vi "ReadSerial_and_Plot_Basic_JE_002.vi"() -> ()   [LabVIEW 2011]
uses:
  <vilib>/Instr/_visa.llb/VISA Configure Serial Port (Serial Instr).vi
panel:
  in  "N data blocks to read":dbl=1.0
  in  "byte order (0:big-endian, network order) 2":T1(ring)
  out "Nbytes written from Teensy to Serial Port":u32
  out "strlen":i32
  in  "byte order (0:big-endian, network order)":T1(ring)
  out "Graphical Representation of 1-D Data Stream":u16[](graph)
  out "concatenated string":string
  out "ascii code u8":i32
  out "Waveform Chart for 32 Chans":T2(graph)
  out "size(s)":i32
  in  "stop":bool
  in  "VISA resource name":refnum<visa-resource-name>
  in  "baud rate (9600)":u32=9600
  in  "data bits (8)":u16=8 min=5 max=8 step=1
  in  "stop bits (10: 1 bit)":u16(ring)=10 items=["1.0"=10, "1.5"=15, "2.0"=20]
  in  "flow control (0:none)":u16(ring) items=["None", "XON/XOFF", "RTS/CTS", "XON/XOFF & RTS/CTS", "DTR/DSR", "XON/XOFF & DTR/DSR"]
  in  "parity (0:none)":enum16{"None", "Odd", "Even", "Mark", "Space"}(ring)
  in  "file (use dialog)":path
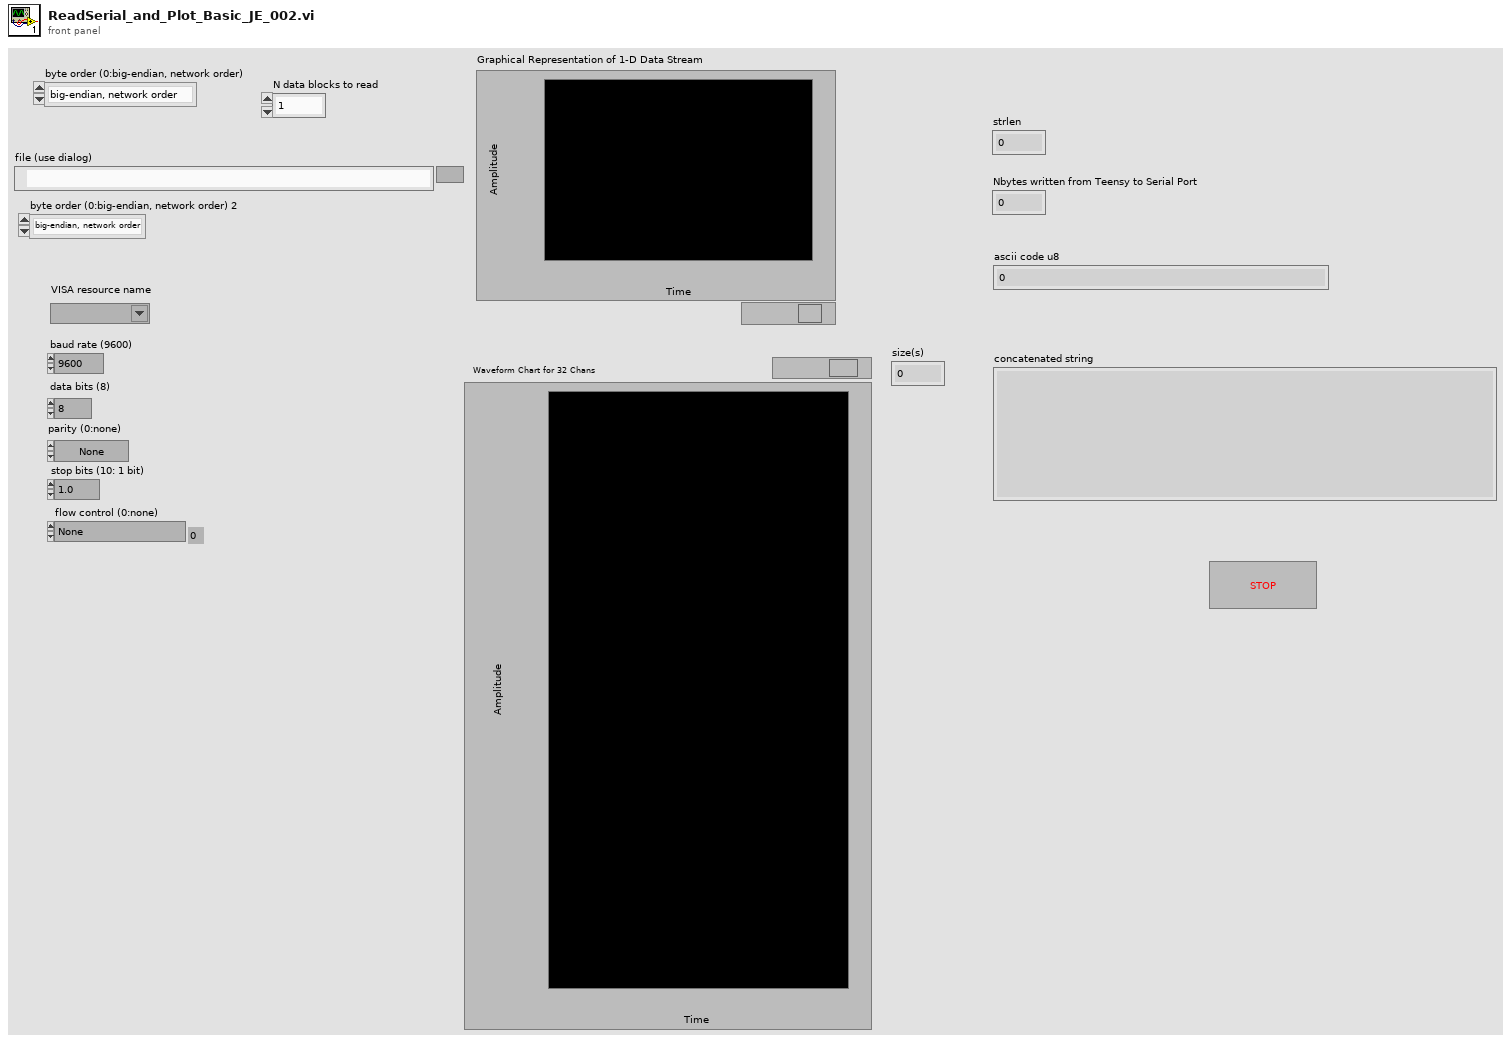
[diagram p1: front panel]
types:
  T1 = enum16{"big-endian, network order", "native, host order", "little-endian"}
  T2 = cluster{"[0]":u16, "[1]":u16, "[2]":u16, "[3]":u16, "[4]":u16, "[5]":u16, "[6]":u16, "[7]":u16, "[8]":u16, "[9]":u16, "[10]":u16, "[11]":u16, "[12]":u16, "[13]":u16, "[14]":u16, "[15]":u16, "[16]":u16, "[17]":u16, "[18]":u16, "[19]":u16, "[20]":u16, "[21]":u16, "[22]":u16, "[23]":u16, "[24]":u16, "[25]":u16, "[26]":u16, "[27]":u16, "[28]":u16, "[29]":u16, "[30]":u16, "[31]":u16}
  T3 = enum16{"open", "replace", "create", "open or create", "replace or create", "replace or create with confirmation"}
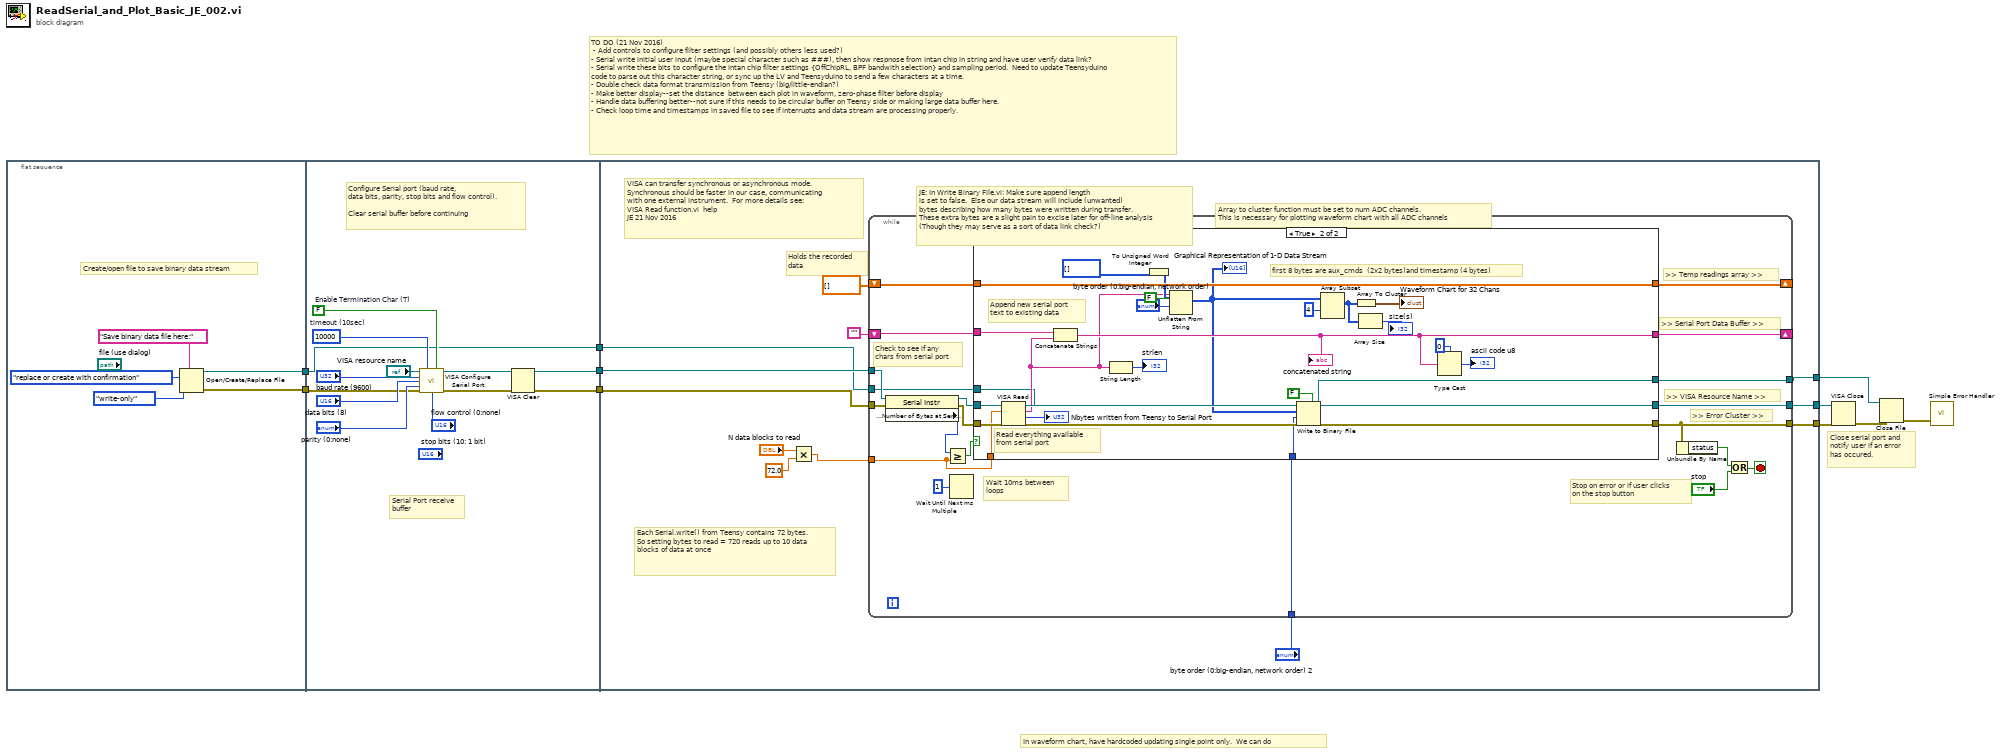
[diagram p0: block diagram]
diagram:
  # "TO DO (21 Nov 2016)\n - Add controls to configure filter settings (and possibly others less used?)\n- Serial write initial user input (maybe special character such as ###), then show respnose from Intan chip in string and have user verify data link?\n- Serial write these bits to configure the Intan chip filter settings {OffChipRL, BPF bandwith selection} and sampling period.  Need to update Teensyduino code to parse out this character string, or sync up the LV and Teensyduino to send a few characters at a time. \n- Double check data format transmission from Teensy (big/little-endian?)\n- Make better display--set the distance  between each plot in waveform, zero-phase filter before display\n- Handle data buffering better--not sure if this needs to be circular buffer on Teensy side or making large data buffer here.\n- Check loop time and timestamps in saved file to see if interrupts and data stream are processing properly."
  # "In waveform chart, have hardcoded updating single point only.  We can do"
  # "Close serial port and\nnotify user if an error\nhas occured."
  n1 = flat-sequence {
    tunnel: [w12] -> w10
    tunnel: [w11] -> w2
    tunnel: w10 -> [w19]
    tunnel: [w18] -> w4
    tunnel: [w17] -> w3
    tunnel: w2 -> [w16]
    tunnel: [w16] -> w1
    tunnel: [w34] -> w7
    tunnel: [w33] -> w6
    tunnel: [w32] -> w5
    tunnel: w4 -> [w31]
    tunnel: w3 -> [w30]
    tunnel: w1 -> [w29]
    frame #0 {
      # "Create/open file to save binary data stream"
      n2 = Open/Create/Replace File(prompt="Save binary data file here:" ("prompt (Choose or enter file path)"), operation (0:open)=T3."replace or create with confirmation", access (0:read/write)=enum16{"read/write", "read-only", "write-only"}."write-only") -> (refnum out=w11:refnum<file>, error out=w12:errorcluster)  [unwired: 3 in, 1 out]
    }
    frame #1 {
      w27 = FALSE  # Enable Termination Char (T)
      w28 = u32 10000  # timeout (10sec)
      # "Configure Serial port (baud rate,\ndata bits, parity, stop bits and flow control).\n\nClear serial buffer before continuing"
      # "Serial Port receive\nbuffer"
      n3 = call-poly "VISA Configure Serial Port"("VISA resource name"="VISA resource name", "timeout (10sec)"=w28, "Enable Termination\nChar (T)"=w27, "baud rate (9600)"="baud rate (9600)", "data bits (8)"="data bits (8)", "parity (0:none)"="parity (0:none)", "error in (no error)"=w19, "flow control (0:none)"="flow control (0:none)") -> ("VISA resource name out"=w25:refnum<visa-resource-name>, "error out"=w26:errorcluster)  [unwired: 6 in]
      n4 = VISA Clear(VISA resource name=w25, error in (no error)=w26) -> (VISA resource name out=w18:refnum<visa-resource-name>, error out=w17:errorcluster)
    }
    frame #2 {
      # "Holds the recorded\ndata"
      # "Each Serial.write() from Teensy contains 72 bytes.  So setting bytes to read = 720 reads up to 10 data blocks of data at once"
      # "Array to cluster function must be set to num ADC channels. \nThis is necessary for plotting waveform chart with all ADC channels"
      # "JE: In Write Binary File.vi: Make sure append length \nis set to false.  Else our data stream will include (unwanted)\nbytes describing how many bytes were written during transfer.\nThese extra bytes are a slight pain to excise later for off-line analysis\n(Though they may serve as a sort of data link check?)"
      # "VISA can transfer synchronous or asynchronous mode.\nSynchronous should be faster in our case, communicating\nwith one external instrument.  For more details see: \nVISA Read function.vi  help \nJE 21 Nov 2016"
      n5 = Multiply(x="N data blocks to read", y=72.0) -> (x*y=w35:dbl)
      n6 = while {
        tunnel: [w55] -> w32
        tunnel: [w60] -> w33
        shift-right: [w49] -> _
        shift-left: "" -> [w57]
        shift-right: [w51] -> _
        shift-left: dbl[] [] -> [w50]
        tunnel: [w46] -> w34
        tunnel: "byte order (0:big-endian, network order) 2" -> [w45]
        tunnel: w35 -> [w44]
        tunnel: w31 -> [w43]
        tunnel: w30 -> [w42]
        tunnel: w29 -> [w41]
        stop <- w54 stop-if-true
        # "Wait 10ms between \nloops"
        # "Stop on error or if user clicks \non the stop button"
        # ">> Error Cluster >>"
        # ">> VISA Resource Name >>"
        # ">> Temp readings array >>"
        # ">> Serial Port Data Buffer >>"
        # "Check to see if any\nchars from serial port"
        n7 = property class="Serial Instr"(reference=w43, error in=w42) -> (reference out=w59:refnum<visa-resource-name>, error out=w58:errorcluster, "Serial Settings:Number of Bytes at Serial Port"=w48:u32)
        n8 = Greater Or Equal?(x=w48, y=w44) -> (x >= y?=w47:bool)
        n9 = Wait Until Next ms Multiple(millisecond multiple=u32 1) -> ()  [unwired: 1 out]
        n10 = case shown="True" w47 {
          tunnel: [w64 w77] -> w55
          tunnel: [w65 w92] -> w60
          tunnel: w59 -> [w65 w91]
          tunnel: w58 -> [w64 w90]
          tunnel: w57 -> [w63 w89]
          tunnel: [w63 w83] -> w49
          tunnel: [w62 w86] -> w51
          tunnel: w50 -> [w62 w86]
          tunnel: w44 -> [_ w88]
          tunnel: [w61 w76] -> w46
          tunnel: w45 -> [_ w72]
          tunnel: w41 -> [w61 w66]
          frame False {
            # "No data in from serial port - Nothing to do."
          }
          frame True {
            # "first 8 bytes are aux_cmds  (2x2 bytes)and timestamp (4 bytes)"
            # "Append new serial port\ntext to existing data"
            # "Read everything available\nfrom serial port"
            n11 = VISA Read(VISA resource name=w91, byte count=w88, error in (no error)=w90) -> (VISA resource name out=w92:refnum<visa-resource-name>, read buffer=w79:string, return count=→"Nbytes written from Teensy to Serial Port":u32, error out=w78:errorcluster)
            n12 = Concatenate Strings(w89, w79) -> (w83:string)
            "concatenated string" <- w83
            n13 = String Length(string=w79) -> (length=→"strlen":i32)
            n14 = To Unsigned Word Integer(number=i16[] []) -> (unsigned 16bit integer=w80:u16[])
            n15 = Unflatten From String(type=w80, binary string=w79, data includes array or string size? (T)=FALSE, byte order (0:big-endian, network order)="byte order (0:big-endian, network order)") -> (value=w71:u16[])  [unwired: 1 in, 2 out]
            "Graphical Representation of 1-D Data Stream" <- w71
            n16 = Write to Binary File(file (use dialog)=w66, data=w71, error in=w78, 5:FALSE ("prepend array or string size? (T)"), 9:w72) -> (refnum out=w76:refnum<file>, error out=w77:errorcluster)  [unwired: 1 in, 1 out]
            n17 = Array Subset(array=w71, index=4) -> (w68:u16[])  [unwired: 1 in]
            n18 = Array To Cluster(array=w68) -> (cluster=→"Waveform Chart for 32 Chans":T2)
            n19 = Array Size(array=w68) -> (size(s)=→"size(s)":i32)
            n20 = Type Cast(type=0, x=w83) -> (*(type *) &x=→"ascii code u8":i32)
          }
        }
        n21 = Unbundle By Name(w55) -> ("status"=w53:bool)
        n22 = Or(x=w53, y="stop") -> (x .or. y?=w54:bool)
      }
    }
  }
  n23 = VISA Close(VISA resource name=w6, error in (no error)=w5) -> (error out=w9:errorcluster)
  n24 = Close File(refnum=w7, error in=w9) -> (error out=w8:errorcluster)  [unwired: 1 out]
  n25 = call <vilib>:"Simple Error Handler.vi"("error in (no error)"=w8) -> ()  [unwired: 4 in, 5 out]
